vi "sub vi - reset jig cycle v1.vi"() -> ()   [LabVIEW 2013]
panel:
  out "Input Cluster":T1
  in  "value":dbl
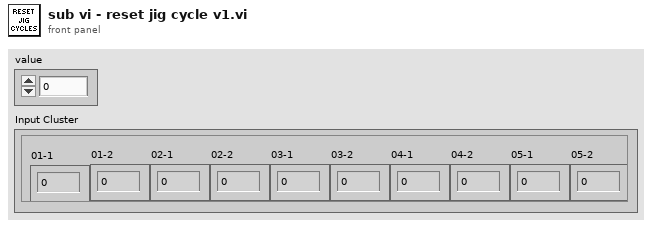
[diagram p1: front panel]
types:
  T1 = cluster{"01-1":dbl, "01-2":dbl, "02-1":dbl, "02-2":dbl, "03-1":dbl, "03-2":dbl, "04-1":dbl, "04-2":dbl, "05-1":dbl, "05-2":dbl}
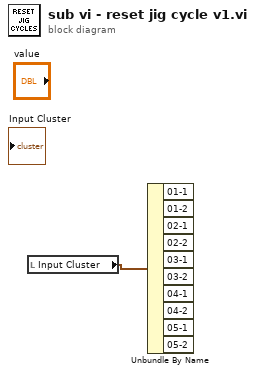
[diagram p0: block diagram]
diagram:
  n1 = local read "Input Cluster"() -> (w1:T1)
  n2 = Unbundle By Name(w1) -> ()  [unwired: 10 out]
